vi "ADS1015_Start_Convert.vi"(7 "I2C Slave Address (0)":u8, 8 "error in (no error)":errorcluster, 9 "I2C_Channel_platform":T1, 10 "Scale mV":u16=2, 11 "LINX Resource in":T2) -> (0 "error out":errorcluster, 2 "mV_out":u16, 3 "LINX Resource out":T2)   [LabVIEW 2014]
uses:
  <vilib>/MakerHub/LINX/Private/Type Defs/LINX Ref.ctl
  <vilib>/MakerHub/LINX/Private/Type Defs/Platform.ctl
  <vilib>/MakerHub/LINX/Private/Type Defs/Interface.ctl
  <vilib>/MakerHub/LINX/Private/Device/Type Defs/LINX Device Config.ctl
  <vilib>/MakerHub/LINX/Private/Device/Type Defs/TCP Config.ctl
  <vilib>/MakerHub/LINX/Private/Device/Type Defs/Channels.ctl
  User Defined/I2C_Platform_Selector.ctl
  <vilib>/MakerHub/LINX/Private/Local IO/LinxI2cWrite.vi
  <vilib>/MakerHub/LINX/Public/Utilities/Check Channel.vi
  <vilib>/MakerHub/LINX/Private/Utilties/Generate Error.vi
  <vilib>/MakerHub/LINX/LMH-LINX.lvlib
  <vilib>/MakerHub/LINX/Private/Device/Device.lvlib
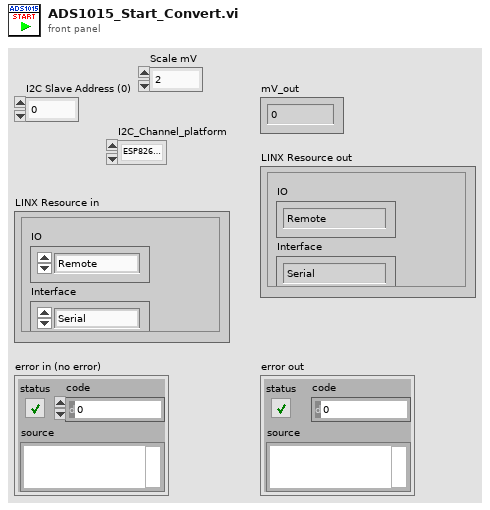
[diagram p1: front panel]
types:
  T1 = typedef "I2C_Platform_Selector.ctl" = enum16{"ESP8266-I2C", "Raspberry Pi-I2C"}
  T2 = typedef "LMH-LINX.lvlib/LINX Ref.ctl" = cluster{"IO":T3, "Interface":T4, "LINX Device Config":T5}
  T3 = typedef "LMH-LINX.lvlib/Platform.ctl" = enum16{"Remote", "Local"}
  T4 = typedef "LMH-LINX.lvlib/Interface.ctl" = enum16{"Serial", "TCP"}
  T5 = typedef "LMH-LINX.lvlib/Device.lvlib/LINX Device Config.ctl" = cluster{"Interface":T4, "COM Port":refnum<visa-resource-name>, "TCP Configuration":T6, "Device Family":u8, "Device ID":u8, "Device Name":string, "TCP Ref":refnum<k5>, "Channels":T7}
  T6 = typedef "LMH-LINX.lvlib/Device.lvlib/TCP Config.ctl" = cluster{"IP Address":string, "Port":u16}
  T7 = typedef "LMH-LINX.lvlib/Channels.ctl" = cluster{"DI":u8[], "DO":u8[], "AI":u8[], "AO":u8[], "PWM":u8[], "QE":u8[], "UART":u8[], "I2C 2":u8[], "SPI":u8[], "CAN":u8[], "Servo":u8[], "AI Ref (V)":dbl, "AI Resolution (Bits)":u8, "AO Ref (V)":dbl, "AO Resolution (Bits)":u8}
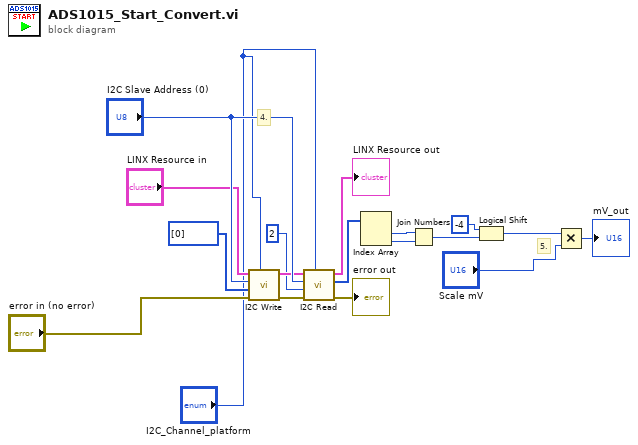
[diagram p0: block diagram]
diagram:
  # "5."
  # "4."
  n1 = call <vilib>:"I2C Write.vi"("I2C Channel"="I2C_Channel_platform", "Error In"="error in (no error)", "Data"=u8[] [0], "I2C Slave Address (0)"="I2C Slave Address (0)", "LINX Resource"="LINX Resource in") -> ("Error Out"=w17:errorcluster, "LINX Resource"=w13:T2)  [unwired: 5 in]
  n2 = call <vilib>:"I2C Read.vi"("I2C Channel"="I2C_Channel_platform", "Error In"=w17, "Bytes To Read"=u8 2, "I2C Slave Address (0)"="I2C Slave Address (0)", "LINX Resource"=w13) -> ("Error Out"=→"error out":errorcluster, "Data"=w10:u8[], "LINX Resource"=→"LINX Resource out":T2)  [unwired: 4 in]
  n3 = Index Array(array=w10) -> (element #1=w7:u8, element #2=w8:u8)  [unwired: 2 in]
  n4 = Join Numbers(hi=w7, lo=w8) -> ((hi.lo)=w6:u16)
  n5 = Logical Shift(y=i8 -4, x=w6) -> (x << y=w12:u16)
  n6 = Multiply(x=w12, y="Scale mV") -> (x*y=→"mV_out":u16)
